vi "Sum_of_Three.vi"() -> ()   [LabVIEW 2025]
panel:
  out "x+y-z":dbl
  in  "z":dbl
  in  "y":dbl
  in  "x":dbl
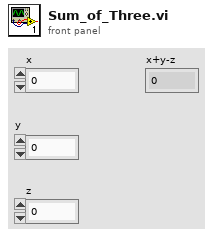
[diagram p1: front panel]
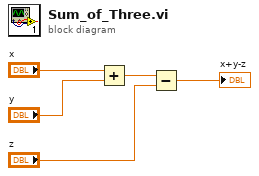
[diagram p0: block diagram]
diagram:
  n1 = Add(x="x", y="y") -> (x+y=w3:dbl)
  n2 = Subtract(x=w3, y="z") -> (x-y=→"x+y-z":dbl)
